vi "WriteVISA_popup.vi"(3 "Command":string, 8 "error in (no error)":errorcluster, 10 "platform":u16(ring) items=["Mac", "PC"], 11 "Input Line Command":string="Write to VISA, \u0000\u0000\u0000\u0010PXI194::0::INSTR, 12") -> (0 "Output Line Command":string, 1 "Cancel":bool, 2 "error out":errorcluster)   [LabVIEW 2020]
panel:
  out "VISA instrument":string
  in  "VISA resource name":refnum<visa-resource-name>="PXI194::0::INSTR"
  in  "Cancel button":bool=TRUE
  in  "OK Button":bool=TRUE
  # "(For serial command add proper terminator \nExample: SOUT 1\\n (turn on output of CS580)."
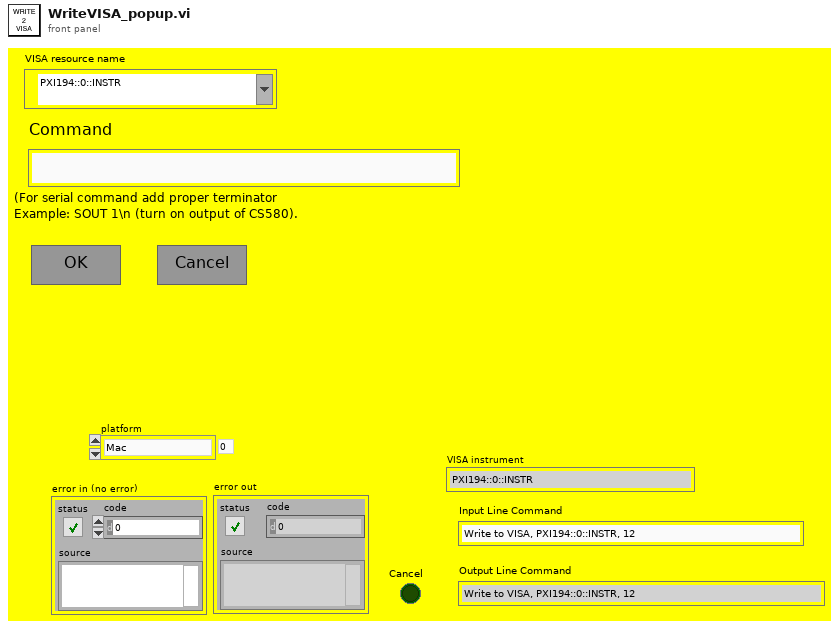
[diagram p1: front panel]
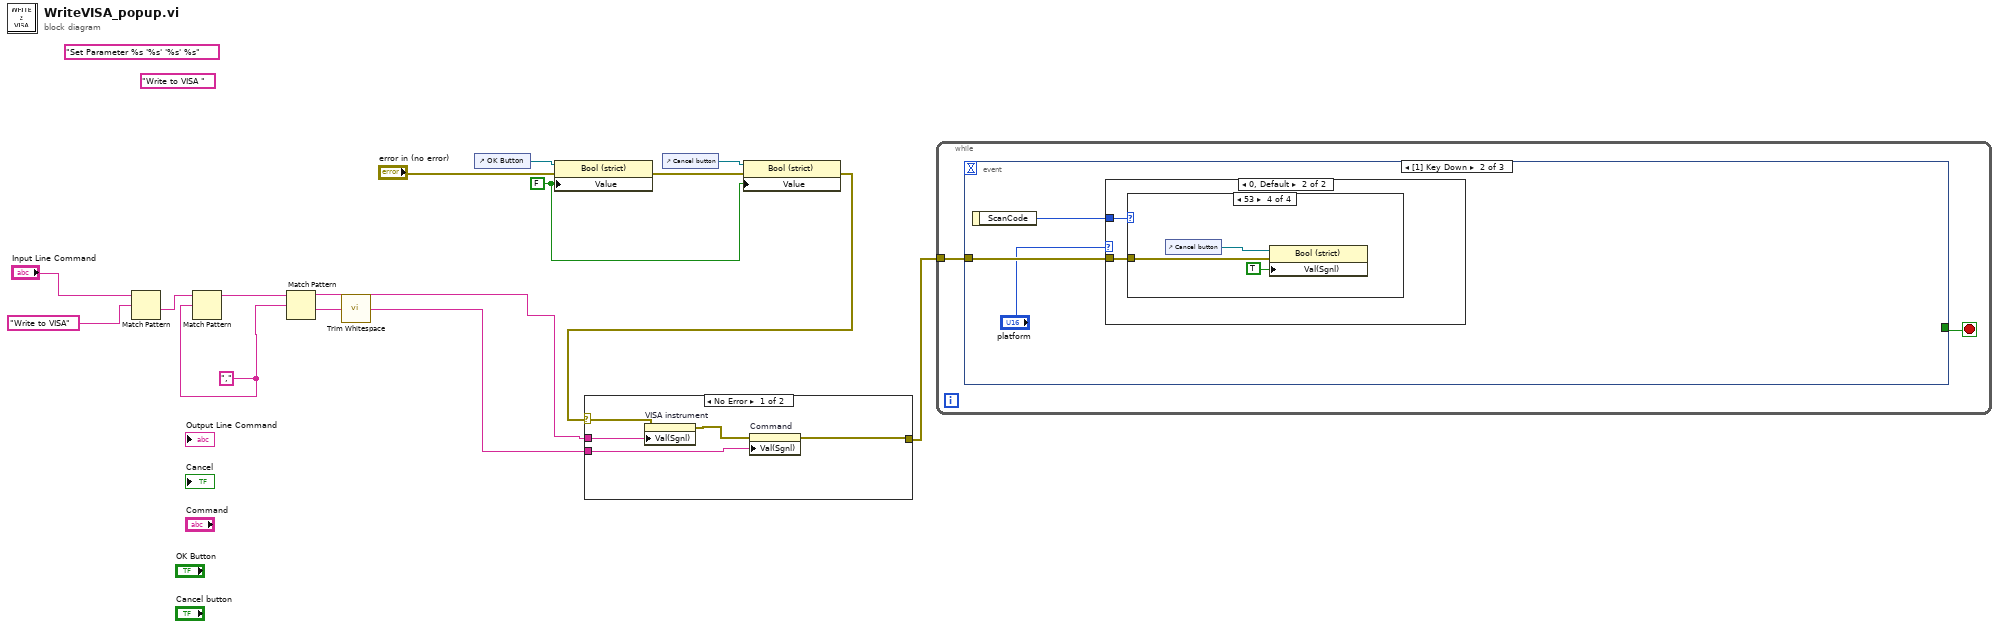
[diagram p0: block diagram]
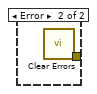
[diagram p2: hidden frame]
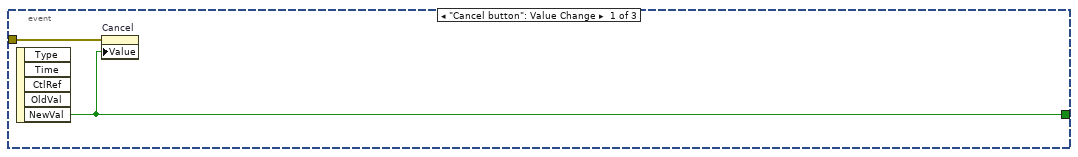
[diagram p3: hidden frame]
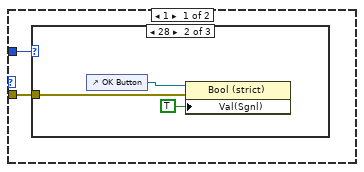
[diagram p4: hidden frame]
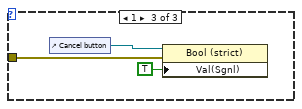
[diagram p6: hidden frame]
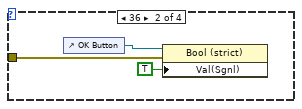
[diagram p8: hidden frame]
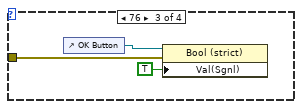
[diagram p9: hidden frame]
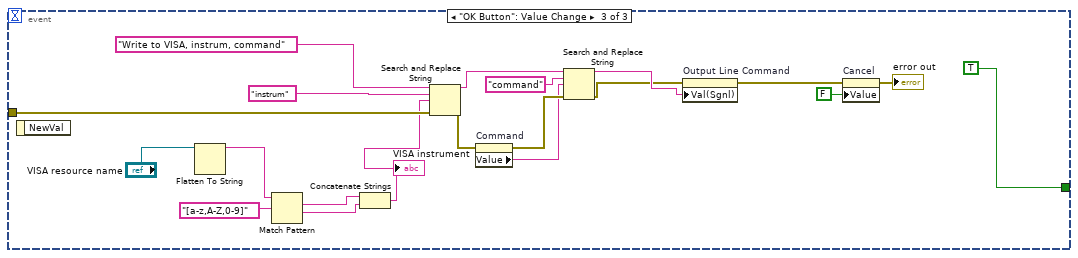
[diagram p10: hidden frame]
diagram:
  (unwired) "Write to VISA " ("format string")
  w4 = "," ("search string/char (-)")
  (unwired) "Set Parameter %s '%s' '%s' %s" ("format string")
  w15 = FALSE
  n1 = Match Pattern(string="Input Line Command", regular expression="Write to VISA" ("search string")) -> (after substring=w6:string)  [unwired: 1 in, 3 out]
  n2 = Match Pattern(string=w6, regular expression=w4) -> (after substring=w5:string)  [unwired: 1 in, 3 out]
  n3 = Match Pattern(string=w5, regular expression=w4) -> (before substring=w3:string, after substring=w2:string)  [unwired: 1 in, 2 out]
  n4 = call <vilib>:"Trim Whitespace.vi"("string"=w2) -> ("trimmed string"=w1:string)  [unwired: 1 in]
  n5 = control-ref of="OK Button"() -> (w14:refnum<vi>)
  n6 = property on="Property Node" class="Bool (strict)"(reference=w14, error in="error in (no error)", "Value"=w15) -> (error out=w11:errorcluster)  [unwired: 1 out]
  n7 = control-ref of="Cancel button"() -> (w13:refnum<vi>)
  n8 = property on="Property Node" class="Bool (strict)"(reference=w13, error in=w11, "Value"=w15) -> (error out=w9:errorcluster)  [unwired: 1 out]
  n9 = case shown="No Error" w9 {
    selector: w9 -> [w16 _]
    tunnel: [w17 w21] -> w10
    tunnel: w3 -> [w20 _]
    tunnel: w1 -> [w19 _]
    frame No Error {
      n10 = property on="VISA instrument" class="Str"(error in=w16, "Val(Sgnl)"=w20) -> (error out=w18:errorcluster)  [unwired: 1 in, 1 out]
      n11 = property on="Command" class="Str"(error in=w18, "Val(Sgnl)"=w19) -> (error out=w17:errorcluster)  [unwired: 1 in, 1 out]
    }
    frame Error {
      n12 = call <vilib>:"Clear Errors.vi"() -> ("error out"=w21:errorcluster)  [unwired: 6 in, 1 out]
    }
  }
  n13 = while {
    tunnel: w10 -> [w23]
    stop <- w22 stop-if-true
    n14 = event shown="[1] Key Down" {
      selector: _ -> [_ _ _]
      dyn-events: _ -> [_ _ _]
      timeout: _ -> [_ _ _]
      tunnel: w23 -> [w25 w27 w59]
      tunnel: [w24 _ TRUE] -> w22
      event "Cancel button": Value Change {
        n15 = event-data() -> ("NewVal"=w24:bool)  [unwired: 1 in, 4 out]
        n16 = property on="Cancel" class="Bool (strict)"(error in=w25, "Value"=w24) -> ()  [unwired: 1 in, 2 out]
      }
      event Key Down {
        n17 = event-data() -> ("ScanCode"=w28:i16)  [unwired: 1 in]
        n18 = case shown="0, Default" "platform" {
          tunnel: w28 -> [w30 w38]
          tunnel: w27 -> [w29 w37]
          frame 1 {
            n19 = case shown="28" w30 {
              tunnel: w29 -> [_ w33 w35]
              frame Default {
              }
              frame 28 {
                n20 = control-ref of="OK Button"() -> (w31:refnum<vi>)
                n21 = property on="Property Node" class="Bool (strict)"(reference=w31, error in=w33, "Val(Sgnl)"=TRUE ("Value (Signaling)")) -> ()  [unwired: 2 out]
              }
              frame 1 {
                n22 = control-ref of="Cancel button"() -> (w34:refnum<vi>)
                n23 = property on="Property Node" class="Bool (strict)"(reference=w34, error in=w35, "Val(Sgnl)"=TRUE ("Value (Signaling)")) -> ()  [unwired: 2 out]
              }
            }
          }
          frame 0, Default {
            n24 = case shown="53" w38 {
              tunnel: w37 -> [_ w41 w44 w46]
              frame Default {
              }
              frame 36 {
                n25 = control-ref of="OK Button"() -> (w39:refnum<vi>)
                n26 = property on="Property Node" class="Bool (strict)"(reference=w39, error in=w41, "Val(Sgnl)"=TRUE ("Value (Signaling)")) -> ()  [unwired: 2 out]
              }
              frame 76 {
                n27 = control-ref of="OK Button"() -> (w42:refnum<vi>)
                n28 = property on="Property Node" class="Bool (strict)"(reference=w42, error in=w44, "Val(Sgnl)"=TRUE ("Value (Signaling)")) -> ()  [unwired: 2 out]
              }
              frame 53 {
                n29 = control-ref of="Cancel button"() -> (w45:refnum<vi>)
                n30 = property on="Property Node" class="Bool (strict)"(reference=w45, error in=w46, "Val(Sgnl)"=TRUE ("Value (Signaling)")) -> ()  [unwired: 2 out]
              }
            }
          }
        }
      }
      event "OK Button": Value Change {
        n31 = event-data() -> ()  [unwired: 1 in, 1 out]
        n32 = Flatten To String(anything="VISA resource name") -> (data string=w49:string)  [unwired: 3 in, 2 out]
        n33 = Match Pattern(string=w49, regular expression="[a-z,A-Z,0-9]") -> (match substring=w52:string, after substring=w51:string)  [unwired: 1 in, 2 out]
        n34 = Concatenate Strings(w52, w51) -> (w48:string)
        "VISA instrument" <- w48
        n35 = Search and Replace String(input string="Write to VISA, instrum, command" ("format string"), search string="instrum", replace string=w48, error in=w59) -> (result string=w58:string, error out=w57:errorcluster)  [unwired: 4 in, 2 out]
        n36 = property on="Command" class="Str"(error in=w57) -> (error out=w63:errorcluster, "Value"=w62:string)  [unwired: 1 in, 1 out]
        n37 = Search and Replace String(input string=w58, search string="command", replace string=w62, error in=w63) -> (result string=w56:string, error out=w55:errorcluster)  [unwired: 4 in, 2 out]
        n38 = property on="Output Line Command" class="Str"(error in=w55, "Val(Sgnl)"=w56) -> (error out=w54:errorcluster)  [unwired: 1 in, 1 out]
        n39 = property on="Cancel" class="Bool (strict)"(error in=w54, "Value"=FALSE ("Cancel")) -> (error out=→"error out":errorcluster)  [unwired: 1 in, 1 out]
      }
    }
  }
